vi "Read_From_Serial (SubVI).vi"(7 "error in (no error)":errorcluster, 8 "Event Type":T1 items=["Service Request"=1073684491, "Trigger"=3221168138, "Clear"=1073684493, "VXI Signal"=1073684512, "VXI/VME Interrupt"=3221168161, "VXI/VME Sysfail"=1073684509, "VXI/VME Sysreset"=1073684510, "GPIB CIC"=1073684498, "GPIB Talk"=1073684499, "GPIB Listen"=1073684500, "PXI Interrupt"=1073684514, "Serial Break"=1073684515, "Serial TermChar"=1073684516, "Serial CTS"=1073684521, "Serial DSR"=1073684522, "Serial DCD"=1073684524, "Serial RI"=1073684526, "Serial Character"=1073684533, "USB Interrupt"=1073684535, "All Enabled"=1073709055], 9 "Read Count":u32=1000, 10 "VISA Refnum in":refnum<visa-resource-name>) -> (0 "error out":errorcluster, 2 "read buffer":string, 3 "VISA Refnum out":refnum<visa-resource-name>)   [LabVIEW 2015]
uses:
  <vilib>/Instr/_visa.llb/Select Event Type.ctl
  Test_Code/Global 5.vi
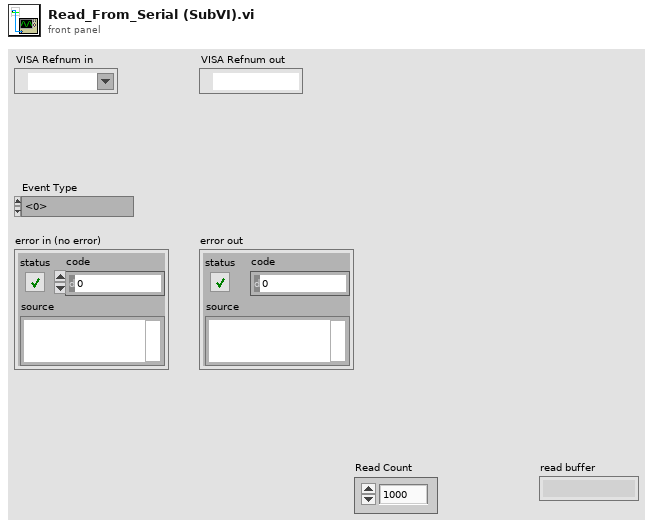
[diagram p1: front panel]
types:
  T1 = typedef "Select Event Type.ctl" = u32
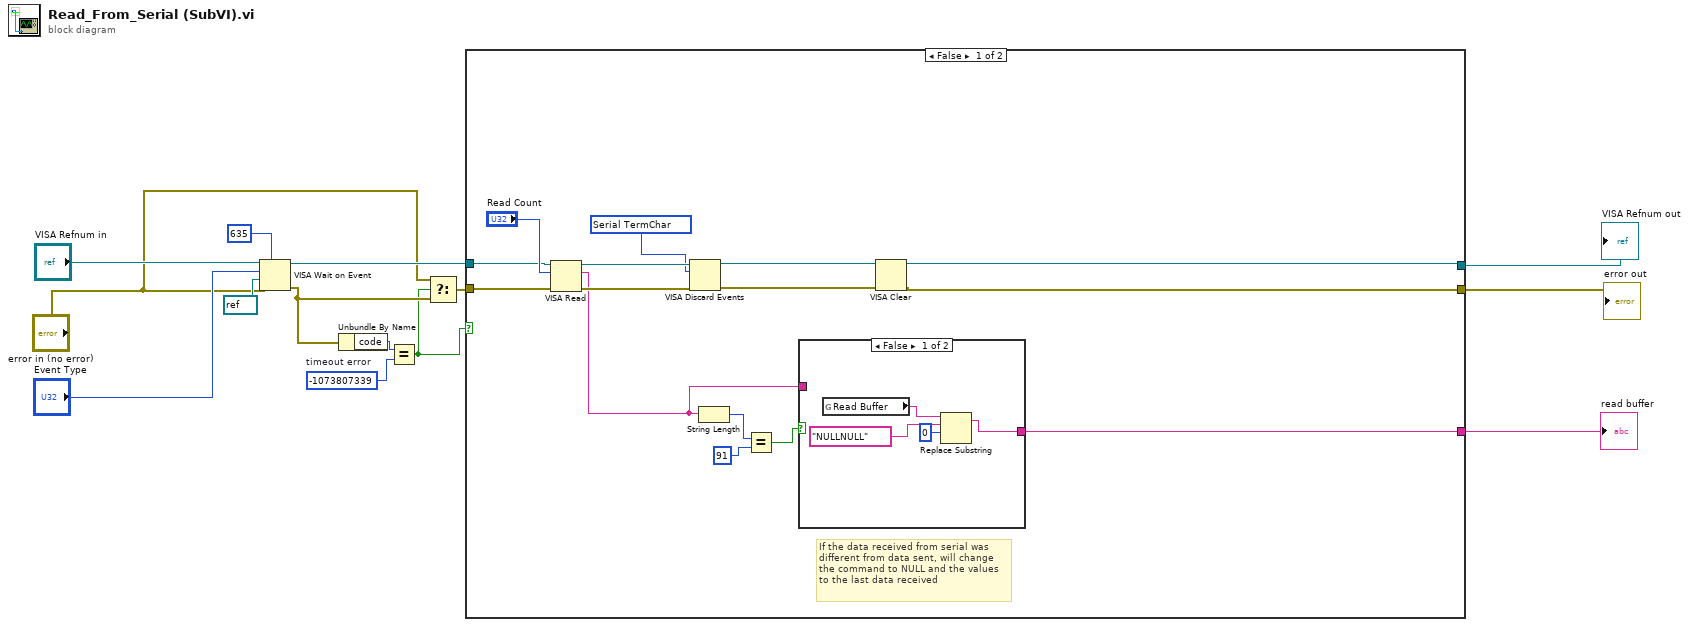
[diagram p0: block diagram]
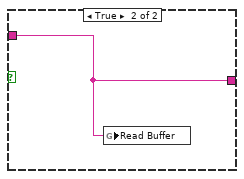
[diagram p2: hidden frame]
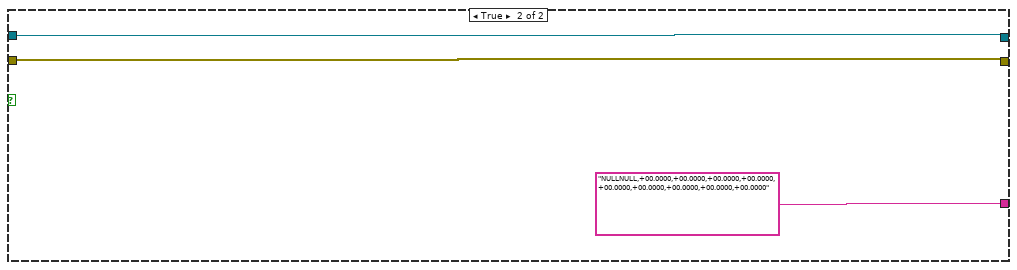
[diagram p3: hidden frame]
diagram:
  w14 = -1073807339  # timeout error
  n1 = VISA Wait on Event(7:u32 635 ("timeout (0)"), 8:"error in (no error)", 9:refnum<visa-resource-name> refnum ("event class (Generic Event)"), 10:"Event Type", 11:"VISA Refnum in") -> (0:w2:errorcluster, 3:w9:refnum<visa-resource-name>)  [unwired: 2 out]
  n2 = Unbundle By Name(w2) -> ("code"=w13:i32)
  n3 = Equal?(x=w13, y=w14) -> (x = y?=w1:bool)
  n4 = Select(t="error in (no error)", s=w1, f=w2) -> (s? t:f=w12:errorcluster)
  n5 = case shown="False" w1 {
    tunnel: w12 -> [w22 w35]
    tunnel: w9 -> [w23 w36]
    tunnel: [w20 w35] -> w6
    tunnel: [w21 w36] -> w5
    tunnel: [w18 "NULLNULL,+00.0000,+00.0000,+00.0000,+00.0000,+00.0000,+00.0000,+00.0000,+00.0000,+00.0000"] -> w3
    frame False {
      w24 = T1 1073684516 items=["Service Request"=1073684491, "Trigger"=3221168138, "Clear"=1073684493, "VXI Signal"=1073684512, "VXI/VME Interrupt"=3221168161, "VXI/VME Sysfail"=1073684509, "VXI/VME Sysreset"=1073684510, "GPIB CIC"=1073684498, "GPIB Talk"=1073684499, "GPIB Listen"=1073684500, "PXI Interrupt"=1073684514, "Serial Break"=1073684515, "Serial TermChar"=1073684516, "Serial CTS"=1073684521, "Serial DSR"=1073684522, "Serial DCD"=1073684524, "Serial RI"=1073684526, "Serial Character"=1073684533, "USB Interrupt"=1073684535, "All Enabled"=1073709055] ("Event Type")
      # "If the data received from serial was different from data sent, will change  the command to NULL and the values to the last data received"
      n6 = VISA Read(VISA resource name=w23, byte count="Read Count", error in (no error)=w22) -> (VISA resource name out=w26:refnum<visa-resource-name>, read buffer=w15:string, error out=w25:errorcluster)  [unwired: 1 out]
      n7 = VISA Discard Events(8:w25, 10:w24, 11:w26) -> (0:w28:errorcluster, 3:w29:refnum<visa-resource-name>)  [unwired: 1 in]
      n8 = String Length(string=w15) -> (length=w17:i32)
      n9 = Equal?(x=w17, y=91 ("x")) -> (x = y?=w19:bool)
      n10 = case shown="False" w19 {
        tunnel: [w33 w34] -> w18
        tunnel: w15 -> [_ w34]
        frame False {
          n11 = global read "Global 5.vi" "Read Buffer"() -> (w32:string)
          n12 = Replace Substring(3:0 ("offset (0)"), 4:"NULLNULL" ("substring (\"\")"), 5:w32) -> (1:w33:string)  [unwired: 1 in, 1 out]
        }
        frame True {
          n13 = global write "Global 5.vi" "Read Buffer"(w34) -> ()
        }
      }
      n14 = VISA Clear(VISA resource name=w29, error in (no error)=w28) -> (VISA resource name out=w21:refnum<visa-resource-name>, error out=w20:errorcluster)
    }
    frame True {
    }
  }
  "VISA Refnum out" <- w5
  "error out" <- w6
  "read buffer" <- w3
